vi "Create.vi"(8 "error in (no error)":errorcluster, 11 "Robot_Interface in":refnum<class "Robot_Interface.lvclass">) -> (0 "error out":errorcluster, 3 "Robot_Interface out":refnum<class "Robot_Interface.lvclass">)   [LabVIEW 2015, in "Robot_Interface.lvclass"]
uses:
  Robot_Interface.lvclass
  Subsytems/JKI.Robot.SMO/JKI.Robot.SMO.lvclass
  Robot_Interface.lvclass/Robot_Interface.ctl
  <vilib>/JKI/JKI SMO/SMO/SMO.lvclass
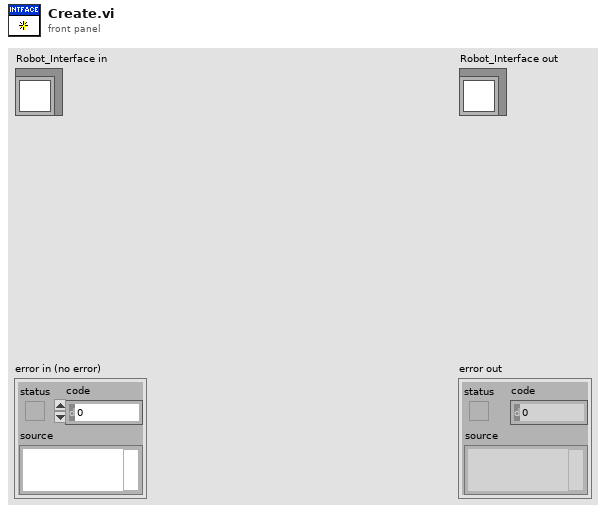
[diagram p1: front panel]
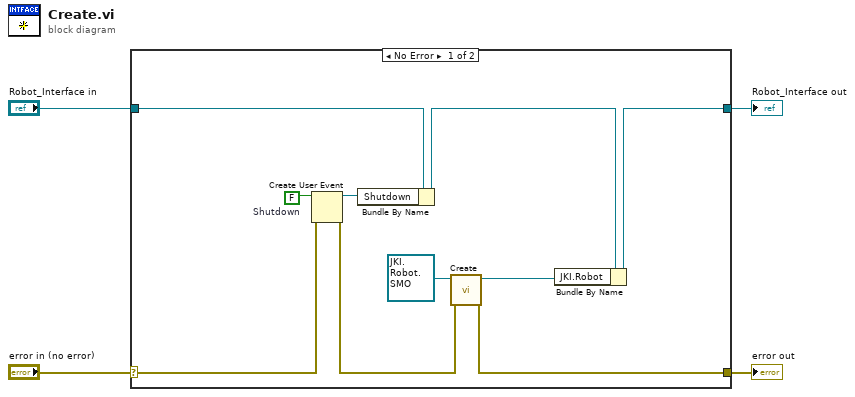
[diagram p0: block diagram]
diagram:
  n1 = case shown="No Error" "error in (no error)" {
    selector: "error in (no error)" -> [w11 w16]
    tunnel: [w8 w16] -> w3
    tunnel: [w6 w15] -> w1
    tunnel: "Robot_Interface in" -> [w12 w15]
    frame No Error {
      w14 = FALSE  # Shutdown
      n2 = Create User Event(user event datatype=w14, error in=w11) -> (user event=w13:refnum<user-event>, error out=w9:errorcluster)
      n3 = Bundle By Name(cluster=w12, "Shutdown"=w13) -> (w7:refnum<class "Robot_Interface.lvclass">)
      n4 = call <vilib>:"Create.vi"("error in (no error)"=w9, "SMO"=refnum<class "JKI.Robot.SMO.lvclass"> refnum ("SMO.Template.lvclass")) -> ("error out"=w8:errorcluster, "SMO out"=w5:refnum<class "JKI.Robot.SMO.lvclass">)  [unwired: 7 in, 1 out]
      n5 = Bundle By Name(cluster=w7, "JKI.Robot"=w5) -> (w6:refnum<class "Robot_Interface.lvclass">)
    }
    frame Error {
    }
  }
  "error out" <- w3
  "Robot_Interface out" <- w1
